vi "Sort File Paths.vi"(11 "File Paths":path[](array[path])) -> (3 "Sorted File Paths":path[](array[path]))   [LabVIEW 2023, in "VIDoc Parsing.lvlib" / "VIDoc Parser.lvclass"]
uses:
  VIDoc Parser.lvclass
  VIDoc Parser.lvclass/VIDoc Parser.ctl
  <vilib>/Utility/miscctls.llb/LVMapReplaceAction.ctl
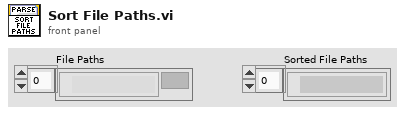
[diagram p1: front panel]
types:
  T1 = typedef "LVMapReplaceAction.ctl" = enum32{"Modify Entry only if found", "Add or Modify Entry", "Delete Entry"}
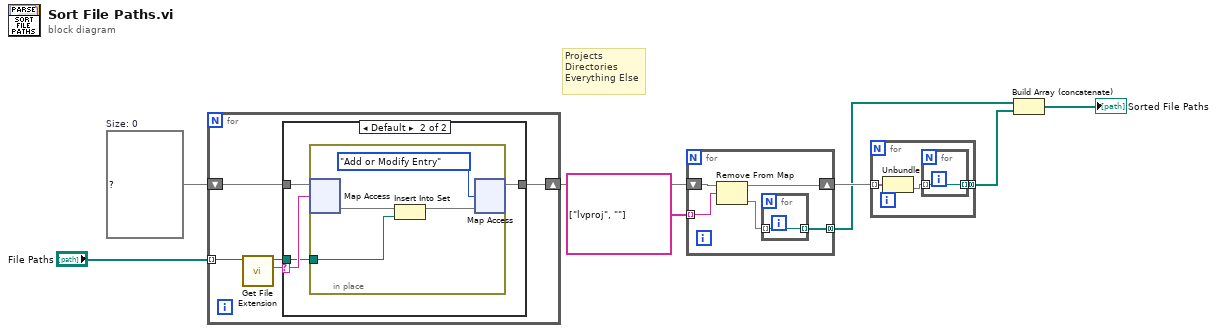
[diagram p0: block diagram]
diagram:
  w7 = map{string, set{path}} {}  # Size: 0
  # "Projects\nDirectories\nEverything Else"
  n1 = for {
    tunnel: "File Paths" -> [w13] mode=indexing
    shift-right: [w9] -> w3
    shift-left: w7 -> [w12]
    n2 = call <vilib>:"Get File Extension.vi"("file"=w13) -> ("lowercase file extension"=w11:string, "dup file"=w10:path)  [unwired: 6 in, 3 out]
    n3 = case shown="Default" w11 {
      selector: w11 -> [_ w17]
      tunnel: w12 -> [w14 w18]
      tunnel: w10 -> [_ w16]
      tunnel: [w14 w15] -> w9
      frame ".git", "git" {
        # "Ignore the .git folder"
      }
      frame Default {
        n4 = in-place {
          in-place-border: w16 -> [w19]
          n5 = in-place-map #1(w18, w17) -> (w21:set{path})  [unwired: 1 in, 1 out]
          n6 = Insert Into Set(10:w19, 11:w21) -> (3:w20:set{path})  [unwired: 1 out]
          n7 = in-place-map #1(w20, LVMapReplaceAction."Add or Modify Entry" ("action")) -> (w15:map{string, set{path}})  [unwired: 2 out]
        }
      }
    }
  }
  n8 = for {
    tunnel: string[] ["lvproj", ""] -> [w25] mode=indexing
    shift-right: [w26] -> w2
    shift-left: w3 -> [w27]
    tunnel: [w23] -> w1 mode=concatenating
    n9 = Remove From Map(10:w25, 11:w27) -> (1:w24:set{path}, 3:w26:map{string, set{path}})  [unwired: 1 out]
    n10 = for {
      tunnel: [w28] -> w23 mode=indexing
      tunnel: w24 -> [w28] mode=indexing
    }
  }
  n11 = for {
    tunnel: w2 -> [w31] mode=indexing
    tunnel: [w29] -> w6 mode=concatenating
    n12 = Unbundle(w31) -> (w30:set{path})  [unwired: 1 out]
    n13 = for {
      tunnel: [w32] -> w29 mode=indexing
      tunnel: w30 -> [w32] mode=indexing
    }
  }
  n14 = Build Array (concatenate)(w1, w6) -> (→"Sorted File Paths":path[])
